vi "Tests.vi"   [LabVIEW 2024, in "ECU InterComm.lvlib"]
uses:
  ECU InterComm.lvlib
  Queues - Get.vi
  Notifiers - Destroy.vi
  Queues - Destroy.vi
  Queues - Create.vi
  Notifiers - Create.vi
  Notifiers - Get.vi
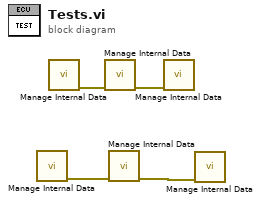
[diagram p0: block diagram]
diagram:
  n1 = call-poly "Manage Internal Data.vi"() -> ("error out"=w2:errorcluster)  [unwired: 11 in]
  n2 = call-poly "Manage Internal Data.vi"() -> ("error out"=w3:errorcluster)  [unwired: 11 in]
  n3 = call-poly "Manage Internal Data.vi"("error in"=w3) -> ("error out"=w4:errorcluster)  [unwired: 9 in, 1 out]
  n4 = call-poly "Manage Internal Data.vi"("error in"=w2) -> ("error out"=w1:errorcluster)  [unwired: 9 in, 1 out]
  n5 = call-poly "Manage Internal Data.vi"("error in"=w4) -> ()  [unwired: 10 in, 1 out]
  n6 = call-poly "Manage Internal Data.vi"("error in"=w1) -> ()  [unwired: 10 in, 1 out]
